vi "Filter Events.vi"(0 "Error":bool, 4 "Warning":bool, 6 "Info":bool, 8 "Debug":bool, 9 "Text Filter":string, 11 "Events":T1[](array[typedef])) -> (3 "Filtered Events":T1[](array[typedef]))   [LabVIEW 2020, in "Volatus.lvlib" / "Event Reporter Module.lvclass"]
uses:
  Event Reporter Module.lvclass
  Event Reporter Module.lvclass/Event Reporter Module.ctl
  Event Element.ctl
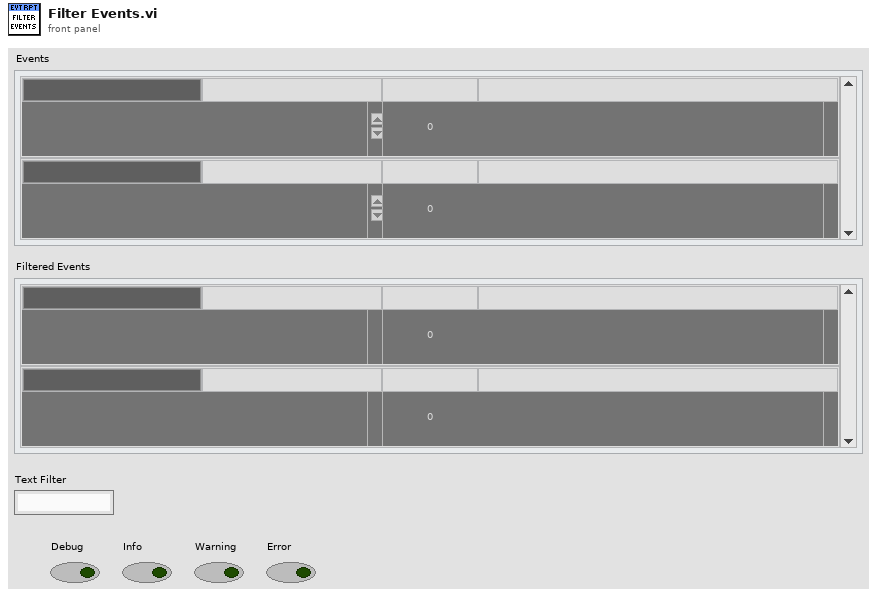
[diagram p1: front panel]
types:
  T1 = typedef "Volatus.lvlib/Event Reporter Module.lvclass/Event Element.ctl" = cluster{"Node":string, "Node Color":u32, "Timestamp":string, "TS Color":u32, "Level":string, "Level Color":u32, "Context":string, "Context Color":u32, "Message":string, "Error Code":i32, "Error Source":string}
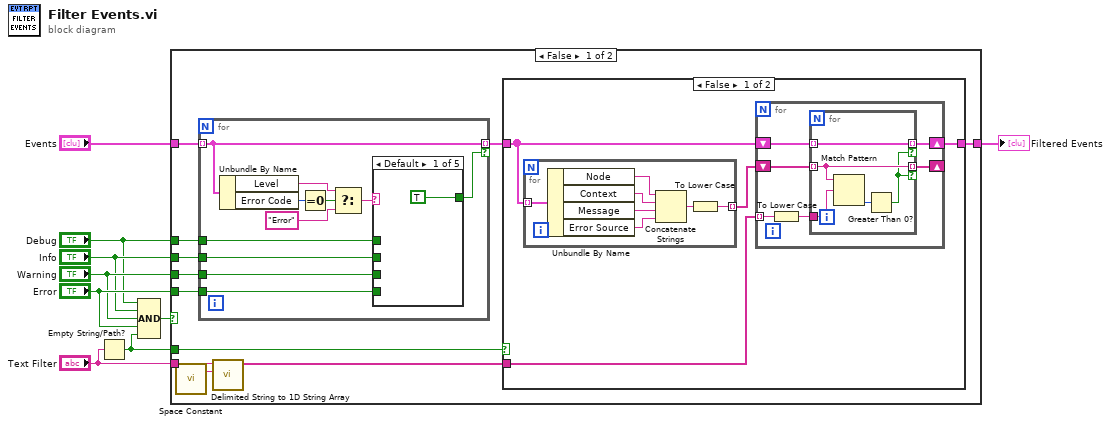
[diagram p0: block diagram]
diagram:
  n1 = Empty String/Path?(string/path="Text Filter") -> (empty?=w1:bool)
  n2 = Compound Arithmetic op=AND("Debug", "Info", "Warning", "Error", w1) -> (w9:bool)
  n3 = case shown="False" w9 {
    tunnel: "Error" -> [w16 _]
    tunnel: "Warning" -> [w17 _]
    tunnel: "Info" -> [w18 _]
    tunnel: "Debug" -> [w19 _]
    tunnel: "Text Filter" -> [w12 _]
    tunnel: [w14 w60] -> w3
    tunnel: "Events" -> [w20 w60]
    tunnel: w1 -> [w15 _]
    frame False {
      n4 = call <vilib>:"Space Constant.vi"() -> ("String"=w11:string)
      n5 = for {
        tunnel: w20 -> [w45] mode=indexing
        tunnel: w19 -> [w49]
        tunnel: w18 -> [w48]
        tunnel: w17 -> [w47]
        tunnel: w16 -> [w46]
        tunnel: [w45] -> w13 mode=indexing if=w44
        n6 = Unbundle By Name(w45) -> ("Level"=w52:string, "Error Code"=w54:i32)
        n7 = Equal To 0?(x=w54) -> (x = 0?=w53:bool)
        n8 = Select(t=w52, s=w53, f="Error") -> (s? t:f=w50:string)
        n9 = case shown="Default" w50 {
          tunnel: w49 -> [_ w56 _ _ _]
          tunnel: w48 -> [_ _ w57 _ _]
          tunnel: w47 -> [_ _ _ w58 _]
          tunnel: w46 -> [_ _ _ _ w59]
          tunnel: [TRUE ("Error") w56 w57 w58 w59] -> w44
          frame Default {
          }
          frame "Debug" {
          }
          frame "Info" {
          }
          frame "Warning" {
          }
          frame "Error" {
          }
        }
      }
      n10 = call <vilib>:"Delimited String to 1D String Array.vi"("delimiter"=w11, "delimited string"=w12) -> ("string array"=w10:string[])  [unwired: 9 in]
      n11 = case shown="False" w15 {
        tunnel: [w22 w43] -> w14
        tunnel: w13 -> [w23 w43]
        tunnel: w10 -> [w21 _]
        frame False {
          n12 = for {
            tunnel: w23 -> [w42] mode=indexing
            tunnel: [w36] -> w24 mode=indexing
            n13 = Unbundle By Name(w42) -> ("Node"=w41:string, "Context"=w40:string, "Message"=w39:string, "Error Source"=w38:string)
            n14 = Concatenate Strings(w41, w40, w39, w38) -> (w37:string)
            n15 = To Lower Case(string=w37) -> (all lower case string=w36:string)
          }
          n16 = for {
            shift-right: [w27] -> _
            shift-left: w24 -> [w29]
            shift-right: [w28] -> w22
            shift-left: w23 -> [w30]
            tunnel: w21 -> [w26] mode=indexing
            n17 = To Lower Case(string=w26) -> (all lower case string=w25:string)
            n18 = for {
              tunnel: w30 -> [w35] mode=indexing
              tunnel: w29 -> [w33] mode=indexing
              tunnel: [w35] -> w28 mode=indexing if=w31
              tunnel: [w33] -> w27 mode=indexing if=w31
              tunnel: w25 -> [w34]
              n19 = Match Pattern(string=w33, regular expression=w34) -> (offset past match=w32:i32)  [unwired: 1 in, 3 out]
              n20 = Greater Than 0?(x=w32) -> (x > 0?=w31:bool)
            }
          }
        }
        frame True {
        }
      }
    }
    frame True {
      # "No filtering"
    }
  }
  "Filtered Events" <- w3
